vi "HK Get Channel Ref.vi"(8 "error in (no error)":errorcluster, 10 "Channel Name":string, 11 "HK Channel in":refnum<class "HK Table.lvclass">) -> (0 "error out":errorcluster, 2 "Channel Ref":refnum<class "HK Item.lvclass">, 3 "HK Channel out":refnum<class "HK Table.lvclass">)   [LabVIEW 2024, in "HK Table.lvclass"]
uses:
  HK Table.lvclass
  HK Item/HK Item.lvclass
  HK Table.lvclass/HK Table.ctl
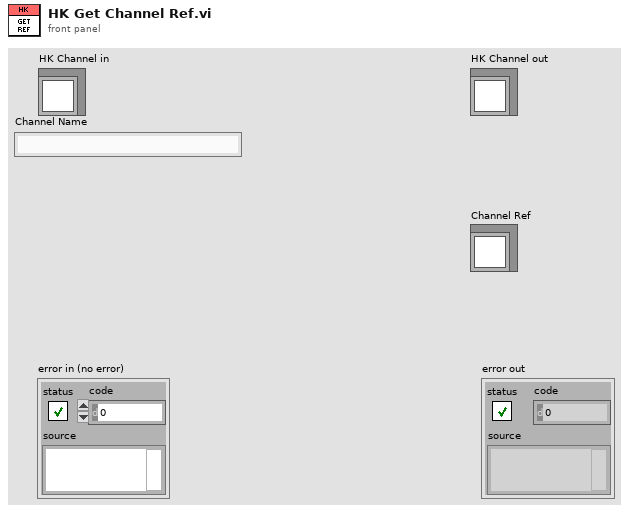
[diagram p1: front panel]
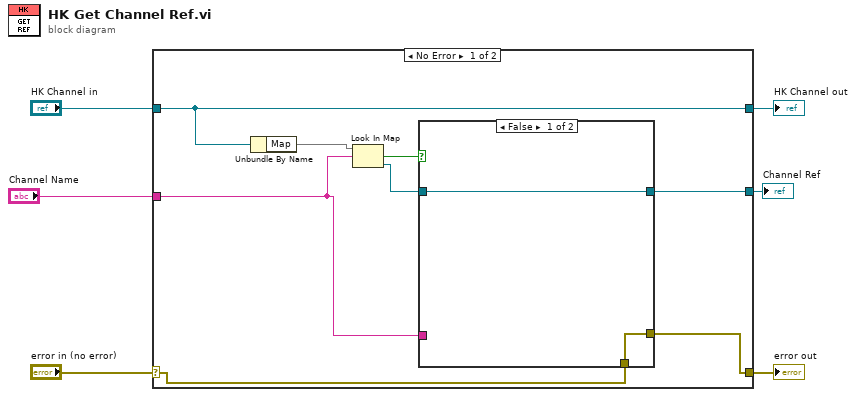
[diagram p0: block diagram]
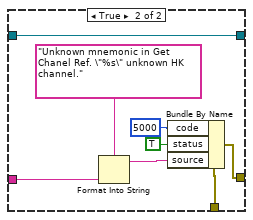
[diagram p2: hidden frame]
diagram:
  n1 = case shown="No Error" "error in (no error)" {
    selector: "error in (no error)" -> [w9 w26]
    tunnel: [w8 w26] -> w5
    tunnel: [w13 w25] -> w3
    tunnel: "HK Channel in" -> [w13 w25]
    tunnel: "Channel Name" -> [w7 _]
    tunnel: [w10 _] -> w1
    frame No Error {
      n2 = Unbundle By Name(w13) -> ("Map"=w14:map{string, refnum<class "HK Item.lvclass">})
      n3 = Look In Map(map=w14, key=w7) -> (key not found?=w12:bool, value=w11:refnum<class "HK Item.lvclass">)  [unwired: 1 in]
      n4 = case shown="False" w12 {
        tunnel: w11 -> [w16 w24]
        tunnel: [w16 w24] -> w10
        tunnel: w9 -> [w15 w19]
        tunnel: [w15 w18] -> w8
        tunnel: w7 -> [_ w17]
        frame False {
        }
        frame True {
          n5 = Format Into String(format string="Unknown mnemonic in Get Chanel Ref. \"%s\" unknown HK channel.", w17) -> (resulting string=w20:string)  [unwired: 2 in, 1 out]
          n6 = Bundle By Name(cluster=w19, "code"=5000, "status"=TRUE, "source"=w20) -> (w18:errorcluster)
        }
      }
    }
    frame Error {
    }
  }
  "error out" <- w5
  "HK Channel out" <- w3
  "Channel Ref" <- w1
